vi "Pot Long Line.vi"(6 "Potting Parameters":T1={"Curing Param A"=0.0, "Curing Param B"=0.0, "Speed Nominal"=-1.0, "Time Nominal"=0.0, "Turn-on Time"=0.0, "Turn-off Time"=0.0, "Safe Height Offset"=0.0, "Tip Height"=0.0, "Width of Line"=0.0, "Number of lines"=1.0, "Distance between lines"=0.0}, 7 "Potting Surface Type":T2, 8 "error in":errorcluster, 9 "End Position":refnum<class "Vec3d Class.lvclass">, 10 "Start Position":refnum<class "Vec3d Class.lvclass">, 11 "SyringeTool in":refnum<class "SyringeTool Class.lvclass">) -> (0 "error out":errorcluster, 3 "SyringeTool out":refnum<class "SyringeTool Class.lvclass">)   [LabVIEW 2017, in "SyringeTool Class.lvclass"]
uses:
  SyringeTool Class.lvclass
  Config Manager Class/Type Definitions/Potting Surface Type.ctl
  Config Manager Class/Type Definitions/Potting Parameters.ctl
  Vec3d Class/Vec3d Class.lvclass
  WorkTable Class/WorkTable Class.lvclass
  Config Manager Class/Config Manager Class.lvclass
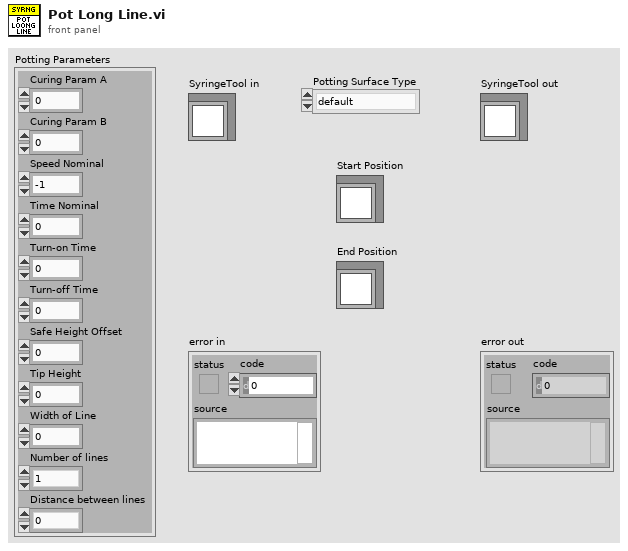
[diagram p1: front panel]
types:
  T1 = typedef "Potting Parameters.ctl" = cluster{"Curing Param A":dbl, "Curing Param B":dbl, "Speed Nominal":dbl, "Time Nominal":dbl, "Turn-on Time":dbl, "Turn-off Time":dbl, "Safe Height Offset":dbl, "Tip Height":dbl, "Width of Line":dbl, "Number of lines":dbl, "Distance between lines":dbl}
  T2 = typedef "Potting Surface Type.ctl" = enum16{"default", "hdi_edge_pads", "bbm_edge_pads", "address_pads"}
  T3 = typedef "Worktable_Syringe.ctl" = cluster{"Syringe Holder":enum16{"Empty", "Populated", "Calibrated"}, "Mixing Time":timestamp, "Tip Offset":refnum<class "Vec3d Class.lvclass">}
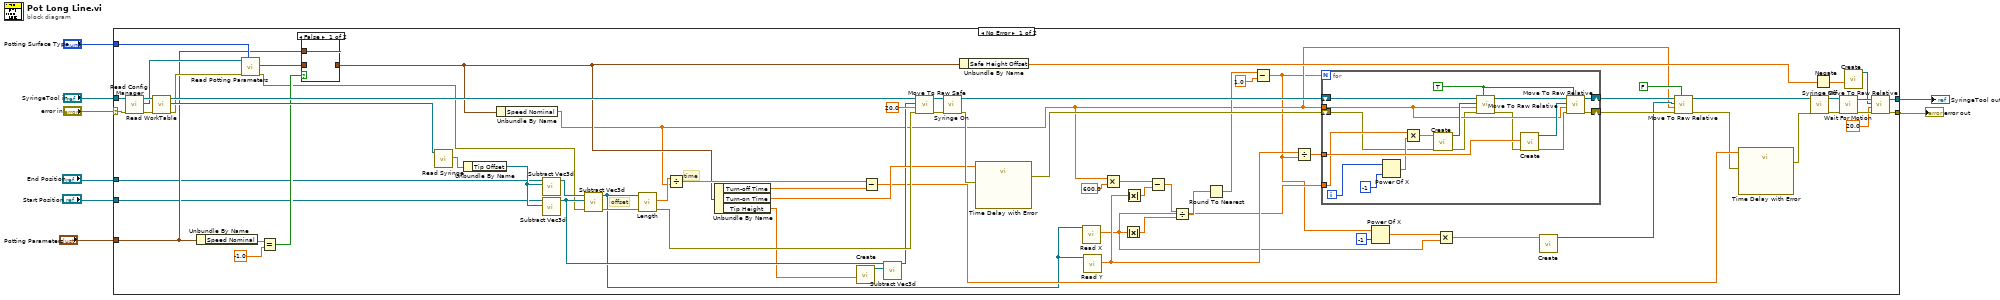
[diagram p0: block diagram]
diagram:
  n1 = case shown="No Error" "error in" {
    selector: "error in" -> [w51 w102]
    tunnel: [w71 w102] -> w7
    tunnel: [w75 w101] -> w5
    tunnel: "SyringeTool in" -> [w59 w101]
    tunnel: "Start Position" -> [w34 _]
    tunnel: "End Position" -> [w35 _]
    tunnel: "Potting Surface Type" -> [w45 _]
    tunnel: "Potting Parameters" -> [w36 _]
    frame No Error {
      # "offset"
      # "time"
      n2 = call-dynamic "Read Config Manager.vi"("error in"=w51, "Gantry in"=w59) -> ("error out"=w53:errorcluster, "Config Manager"=w54:refnum<class "Config Manager Class.lvclass">, "Gantry out"=w58:refnum<class "SyringeTool Class.lvclass">)  [unwired: 7 in]
      n3 = call-dynamic "Read WorkTable.vi"("error in"=w53, "Gantry Class in"=w58) -> ("error out"=w52:errorcluster, "WorkTable Class.lvclass"=w80:refnum<class "WorkTable Class.lvclass">, "Gantry Class out"=w69:refnum<class "SyringeTool Class.lvclass">)  [unwired: 7 in]
      n4 = Unbundle By Name(w36) -> ("Speed Nominal"=w39:dbl)
      n5 = call "Read Potting Parameters.vi"("Potting Surface Type"=w45, "error in"=w52, "Config Manager in"=w54) -> ("error out"=w10:errorcluster, "Potting Parameters"=w40:T1)  [unwired: 6 in, 1 out]
      n6 = Equal?(x=w39, y=-1.0) -> (x = y?=w38:bool)
      n7 = case shown="False" w38 {
        tunnel: w40 -> [_ w100]
        tunnel: [w99 w100] -> w33
        tunnel: w36 -> [w99 _]
        frame False {
        }
        frame True {
        }
      }
      n8 = call "Read Syringe.vi"("WorkTable in"=w80) -> ("Syringe"=w79:T3)  [unwired: 8 in, 2 out]
      n9 = Unbundle By Name(w79) -> ("Tip Offset"=w68:refnum<class "Vec3d Class.lvclass">)
      n10 = Unbundle By Name(w33) -> ("Speed Nominal"=w11:dbl)
      n11 = call "Subtract Vec3d.vi"("Vec3d in 2"=w68, "Vec3d in 1"=w35) -> ("Vec3d Class out"=w70:refnum<class "Vec3d Class.lvclass">)  [unwired: 8 in, 1 out]
      n12 = call "Subtract Vec3d.vi"("Vec3d in 2"=w68, "Vec3d in 1"=w34) -> ("Vec3d Class out"=w48:refnum<class "Vec3d Class.lvclass">)  [unwired: 8 in, 1 out]
      n13 = call "Subtract Vec3d.vi"("error in (no error)"=w10, "Vec3d in 2"=w48, "Vec3d in 1"=w70) -> ("error out"=w67:errorcluster, "Vec3d Class out"=w32:refnum<class "Vec3d Class.lvclass">)  [unwired: 7 in]
      n14 = call-dynamic "Length.vi"("error in"=w67, "Vec3d in"=w32) -> ("error out"=w66:errorcluster, "Length"=w78:dbl)  [unwired: 7 in, 1 out]
      n15 = Divide(x=w78, y=w11) -> (x/y=w77:dbl)
      n16 = Unbundle By Name(w33) -> ("Turn-off Time"=w56:dbl, "Turn-on Time"=w55:dbl, "Tip Height"=w41:dbl)
      n17 = call "Create.vi"("Z"=w41) -> ("Vec3d Class out"=w46:refnum<class "Vec3d Class.lvclass">)  [unwired: 9 in, 1 out]
      n18 = Subtract(x=w77, y=w56) -> (x-y=w44:dbl)
      n19 = call "Subtract Vec3d.vi"("Vec3d in 2"=w46, "Vec3d in 1"=w48) -> ("Vec3d Class out"=w47:refnum<class "Vec3d Class.lvclass">)  [unwired: 8 in, 1 out]
      n20 = call-dynamic "Move To Raw Safe.vi"("error in"=w66, "Speed(mm/s)"=20.0, "Destination"=w47, "Gantry in"=w69) -> ("error out"=w64:errorcluster, "Gantry out"=w63:refnum<class "SyringeTool Class.lvclass">)  [unwired: 6 in]
      n21 = call "Syringe On.vi"("error in"=w64, "SyringeTool"=w63) -> ("error out"=w65:errorcluster, "SyringeTool out"=w76:refnum<class "SyringeTool Class.lvclass">)  [unwired: 8 in]
      n22 = Unbundle By Name(w33) -> ("Safe Height Offset"=w42:dbl)
      n23 = call "Time Delay with Error.vi"("error in (no error)"=w65, "Delay Time (s)"=w55) -> ("error out"=w73:errorcluster)  [unwired: 9 in]
      n24 = call-dynamic "Read X.vi"("Vec3d Class in"=w32) -> ("X"=w13:dbl)  [unwired: 8 in, 2 out]
      n25 = call-dynamic "Read Y.vi"("Vec3d Class in"=w32) -> ("Y"=w24:dbl)  [unwired: 8 in, 2 out]
      n26 = Multiply(x=w11, y=600.0) -> (x*y=w30:dbl)
      n27 = Absolute Value(x=w13) -> (abs(x)=w27:dbl)
      n28 = Absolute Value(x=w24) -> (abs(x)=w29:dbl)
      n29 = Subtract(x=w30, y=w29) -> (x-y=w28:dbl)
      n30 = Divide(x=w28, y=w27) -> (x/y=w26:dbl)
      n31 = Round To Nearest(number=w26) -> (nearest integer value=w16:dbl)
      n32 = Subtract(x=w16, y=1.0) -> (x-y=w9:dbl)
      n33 = Divide(x=w24, y=w9) -> (x/y=w23:dbl)
      n34 = for {
        N: w9 -> [_]
        tunnel: w11 -> [w91]
        shift-right: [w96] -> w21
        shift-left: w76 -> [w98]
        shift-right: [w95] -> w18
        shift-left: w73 -> [w84]
        tunnel: w23 -> [w90]
        tunnel: w13 -> [w88]
        i -> [w85]
        w94 = TRUE ("Wait?")
        n35 = Power Of X(1:-1 ("x"), 2:w85) -> (0:w86:dbl)
        n36 = Multiply(x=w88, y=w86) -> (x*y=w87:dbl)
        n37 = call "Create.vi"("error in"=w84, "X"=w87) -> ("error out"=w83:errorcluster, "Vec3d Class out"=w92:refnum<class "Vec3d Class.lvclass">)  [unwired: 8 in]
        n38 = call-dynamic "Move To Raw Relative.vi"("Wait?"=w94, "error in"=w83, "Speed(mm/s)"=w91, "Delta"=w92, "Gantry in"=w98) -> ("error out"=w82:errorcluster, "Gantry out"=w97:refnum<class "SyringeTool Class.lvclass">)  [unwired: 5 in]
        n39 = call "Create.vi"("error in"=w82, "Y"=w90) -> ("error out"=w81:errorcluster, "Vec3d Class out"=w93:refnum<class "Vec3d Class.lvclass">)  [unwired: 8 in]
        n40 = call-dynamic "Move To Raw Relative.vi"("Wait?"=w94, "error in"=w81, "Speed(mm/s)"=w91, "Delta"=w93, "Gantry in"=w97) -> ("error out"=w95:errorcluster, "Gantry out"=w96:refnum<class "SyringeTool Class.lvclass">)  [unwired: 5 in]
      }
      n41 = Power Of X(1:-1 ("x"), 2:w9) -> (0:w14:dbl)
      n42 = Multiply(x=w14, y=w13) -> (x*y=w15:dbl)
      n43 = call "Create.vi"("X"=w15) -> ("Vec3d Class out"=w12:refnum<class "Vec3d Class.lvclass">)  [unwired: 9 in, 1 out]
      n44 = call-dynamic "Move To Raw Relative.vi"("Wait?"=FALSE, "error in"=w18, "Speed(mm/s)"=w11, "Delta"=w12, "Gantry in"=w21) -> ("error out"=w20:errorcluster, "Gantry out"=w19:refnum<class "SyringeTool Class.lvclass">)  [unwired: 5 in]
      n45 = call "Time Delay with Error.vi"("error in (no error)"=w20, "Delay Time (s)"=w44) -> ("error out"=w43:errorcluster)  [unwired: 9 in]
      n46 = call "Syringe Off.vi"("error in"=w43, "SyringeTool in"=w19) -> ("error out"=w62:errorcluster, "SyringeTool out"=w61:refnum<class "SyringeTool Class.lvclass">)  [unwired: 8 in]
      n47 = Negate(x=w42) -> (-x=w57:dbl)
      n48 = call-dynamic "Wait For Motion.vi"("error in"=w62, "Gantry in"=w61) -> ("error out"=w72:errorcluster, "Gantry out"=w74:refnum<class "SyringeTool Class.lvclass">)  [unwired: 8 in]
      n49 = call "Create.vi"("Z"=w57) -> ("Vec3d Class out"=w60:refnum<class "Vec3d Class.lvclass">)  [unwired: 9 in, 1 out]
      n50 = call-dynamic "Move To Raw Relative.vi"("error in"=w72, "Speed(mm/s)"=20.0, "Delta"=w60, "Gantry in"=w74) -> ("error out"=w71:errorcluster, "Gantry out"=w75:refnum<class "SyringeTool Class.lvclass">)  [unwired: 6 in]
    }
    frame Error {
    }
  }
  "error out" <- w7
  "SyringeTool out" <- w5
